vi "Obtain Request Events.vi"(8 "error in":errorcluster, 10 "Create New? (F)":bool, 11 "Module ID":i32=-1) -> (0 "error out":errorcluster, 2 "Inversor Request Events":T1)   [LabVIEW 2019, in "Inversor.lvlib"]
doc: "This VI Obtains/Creates the Requests events that will be used for other modules to communicate with the module that owns this VI. These Requests events will be accessed only via Public API methods for this module.\n\n<b>NOTE</b>: The contents of this VI are automatically generated and modified by the <b>Tools > DQMH Consortium > DQMH</b> utilities. Consider using those utilities instead of making your own modifications to this VI.\n_____\nBased on DQMH Dev Tools: Project Template 7.1.0.1503."
uses:
  Inversor.lvlib
  Request Events--cluster.ctl
  Stop Argument--cluster.ctl
  Show Panel Argument--cluster.ctl
  Hide Panel Argument--cluster.ctl
  Show Diagram Argument--cluster.ctl
  Get Module Execution Status Argument--cluster.ctl
  Local Instance Request Events--cluster.ctl
  Request Privado Local Argument--cluster.ctl
  Request Privado Argument--cluster.ctl
  Set Voltage Argument--cluster.ctl
  Set Voltage (Reply Payload)--cluster.ctl
  Request Simple Argument--cluster.ctl
  Local Instance Events SEQ/Local Instance Events SEQ.lvlib
panel:
  # "NOTE: The contents of this VI are automatically generated and modified by the Tools > DQMH Consortium > DQMH utilities. Consider using those utilities instead of making your own modifications to this VI."
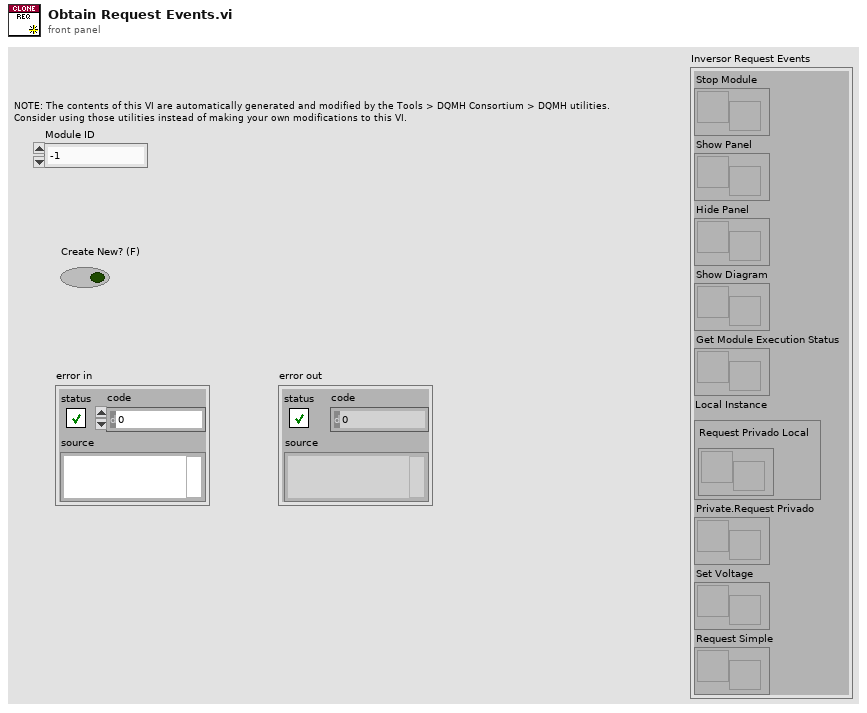
[diagram p1: front panel]
types:
  T1 = typedef "Inversor.lvlib/Request Events--cluster.ctl" = cluster{"Stop Module":refnum<user-event>, "Show Panel":refnum<user-event>, "Hide Panel":refnum<user-event>, "Show Diagram":refnum<user-event>, "Get Module Execution Status":refnum<user-event>, "Local Instance":T2, "Private.Request Privado":refnum<user-event>, "Set Voltage":refnum<user-event>, "Request Simple":refnum<user-event>}
  T2 = typedef "Inversor.lvlib/Local Instance Request Events--cluster.ctl" = cluster{"Request Privado Local":refnum<user-event>}
  T3 = typedef "Inversor.lvlib/Request Simple Argument--cluster.ctl" = cluster{"Module ID":i32, "Numeric":dbl}
  T4 = typedef "Inversor.lvlib/Set Voltage Argument--cluster.ctl" = cluster{"Module ID":i32, "Voltage":dbl, "Wait Notifier":refnum<notifier>, "wait for reply":bool}
  T5 = typedef "Inversor.lvlib/Request Privado Argument--cluster.ctl" = cluster{"Module ID":i32, "String":string}
  T6 = typedef "Inversor.lvlib/Get Module Execution Status Argument--cluster.ctl" = cluster{"Module ID":i32, "Running?":bool}
  T7 = typedef "Inversor.lvlib/Show Diagram Argument--cluster.ctl" = cluster{"Module ID":i32, "Debug?":bool}
  T8 = typedef "Inversor.lvlib/Show Panel Argument--cluster.ctl" = cluster{"Module ID":i32, "Show Panel?":bool}
  T9 = typedef "Inversor.lvlib/Hide Panel Argument--cluster.ctl" = cluster{"Module ID":i32, "Hide Panel?":bool}
  T10 = typedef "Inversor.lvlib/Stop Argument--cluster.ctl" = cluster{"Module ID":i32, "Origin":string, "Exit via Stop Module Req?":bool, "Wait for Module to stop?":bool}
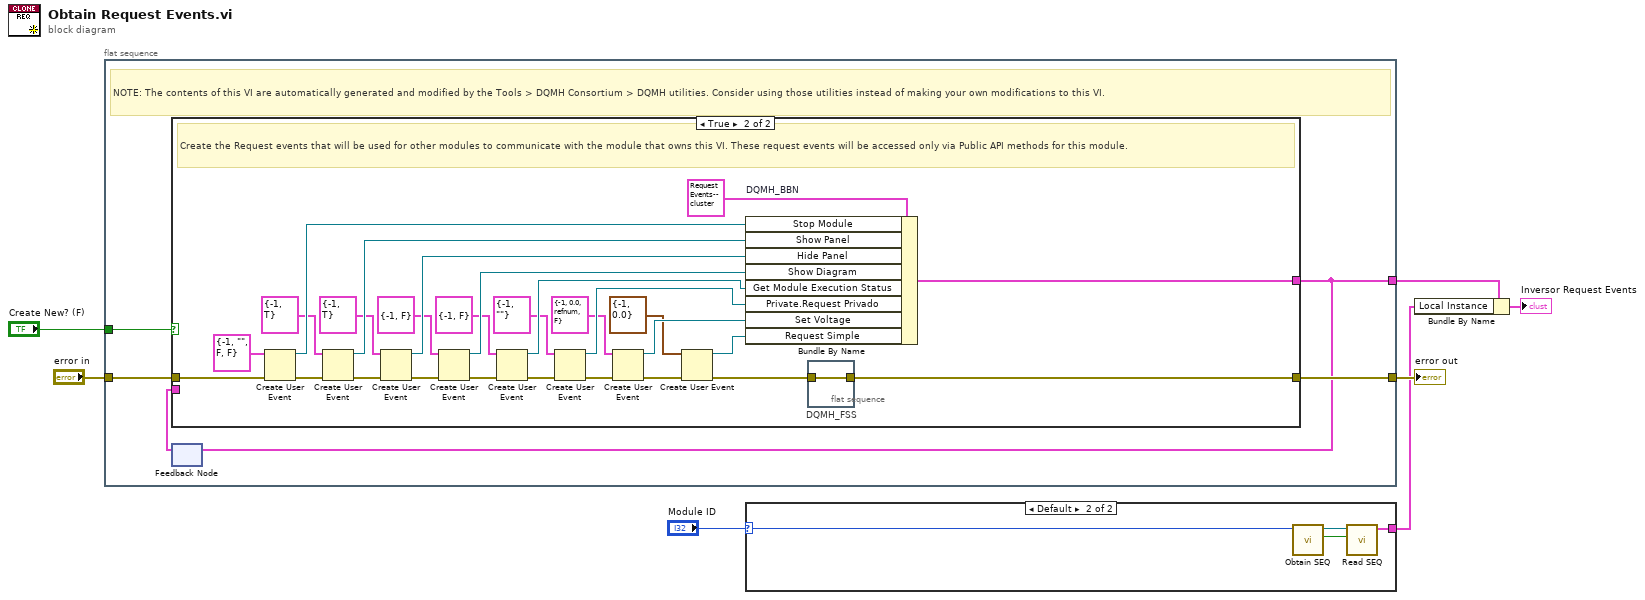
[diagram p0: block diagram]
diagram:
  n1 = flat-sequence {
    tunnel: [w12] -> w7
    tunnel: "error in" -> [w11]
    tunnel: [w9] -> w3
    tunnel: "Create New? (F)" -> [w8]
    frame #0 {
      # "NOTE: The contents of this VI are automatically generated and modified by the Tools > DQMH Consortium > DQMH utilities. Consider using those utilities instead of making your own modifications to this VI."
      n2 = feedback #1() -> (w10:T1)  [unwired: 1 in]
      n3 = case shown="True" w8 {
        tunnel: [w13 w30] -> w12
        tunnel: w11 -> [w13 w42]
        tunnel: [w14 w39] -> w9
        tunnel: w10 -> [w14 _]
        frame False {
        }
        frame True {
          # "Create the Request events that will be used for other modules to communicate with the module that owns this VI. These request events will be accessed only via Public API methods for this module."
          n4 = Create User Event(user event datatype=T10 {"Module ID"=-1, "Origin"="", "Exit via Stop Module Req?"=FALSE, "Wait for Module to stop?"=FALSE} ("Stop Argument"), error in=w42) -> (user event=w40:refnum<user-event>, error out=w37:errorcluster)
          n5 = Create User Event(user event datatype=T8 {"Module ID"=-1, "Show Panel?"=TRUE} ("Show Panel Argument"), error in=w37) -> (user event=w36:refnum<user-event>, error out=w34:errorcluster)
          n6 = Create User Event(user event datatype=T9 {"Module ID"=-1, "Hide Panel?"=TRUE} ("Hide Panel"), error in=w34) -> (user event=w33:refnum<user-event>, error out=w32:errorcluster)
          n7 = Create User Event(user event datatype=T7 {"Module ID"=-1, "Debug?"=FALSE} ("Show Diagram Argument"), error in=w32) -> (user event=w28:refnum<user-event>, error out=w29:errorcluster)
          n8 = Create User Event(user event datatype=T6 {"Module ID"=-1, "Running?"=FALSE} ("Get Module Execution Status Argument"), error in=w29) -> (user event=w25:refnum<user-event>, error out=w26:errorcluster)
          n9 = Create User Event(user event datatype=T5 {"Module ID"=-1, "String"=""} ("Request Privado Argument"), error in=w26) -> (user event=w22:refnum<user-event>, error out=w23:errorcluster)
          n10 = Create User Event(user event datatype=T4 {"Module ID"=-1, "Voltage"=0.0, "Wait Notifier"=refnum, "wait for reply"=FALSE} ("Set Voltage Argument"), error in=w23) -> (user event=w19:refnum<user-event>, error out=w20:errorcluster)
          n11 = Create User Event(user event datatype=T3 {"Module ID"=-1, "Numeric"=0.0} ("Request Simple Argument"), error in=w20) -> (user event=w16:refnum<user-event>, error out=w17:errorcluster)
          n12 = Bundle By Name "DQMH_BBN"(cluster=T1 {"Stop Module"=refnum, "Show Panel"=refnum, "Hide Panel"=refnum, "Show Diagram"=refnum, "Get Module Execution Status"=refnum, "Local Instance"={"Request Privado Local"=refnum}, "Private.Request Privado"=refnum, "Set Voltage"=refnum, "Request Simple"=refnum} ("output cluster"), "Stop Module"=w40, "Show Panel"=w36, "Hide Panel"=w33, "Show Diagram"=w28, "Get Module Execution Status"=w25, "Private.Request Privado"=w22, "Set Voltage"=w19, "Request Simple"=w16) -> (w39:T1)
          n13 = flat-sequence "DQMH_FSS" {
            tunnel: w17 -> [w43]
            tunnel: [w43] -> w30
            frame #0 {
            }
          }
        }
      }
      n14 = feedback-in #1(w9) -> ()
    }
  }
  n15 = case shown="Default" "Module ID" {
    selector: "Module ID" -> [_ w45]
    tunnel: [_ w44] -> w2
    frame -1 {
    }
    frame Default {
      n16 = call "Obtain SEQ.vi"("Module ID"=w45) -> ("Created New?"=w46:bool, "Local Instance Event SEQ"=w47:refnum<queue>)  [unwired: 8 in, 1 out]
      n17 = call "Read SEQ.vi"("Created New?"=w46, "Local Instance Event SEQ"=w47) -> ("Local Instance Request Events"=w44:T2)  [unwired: 8 in, 1 out]
    }
  }
  n18 = Bundle By Name(cluster=w3, "Local Instance"=w2) -> (→"Inversor Request Events":T1)
  "error out" <- w7
